vi "menu options.vi"(8 "error in":errorcluster, 9 "VI ref":refnum<vi>, 11 "menu ref in":refnum<k9>) -> (0 "error out":errorcluster, 3 "menu ref out":refnum<k9>)   [LabVIEW 2013, in "Standard Editor.lvlib"]
uses:
  Standard Editor.lvlib
  <vilib>/Utility/miscctls.llb/LVMenuShortCut.ctl
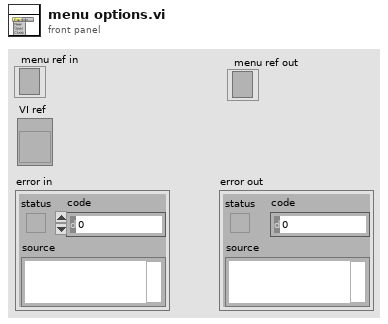
[diagram p1: front panel]
types:
  T1 = typedef "LVMenuShortCut.ctl" = cluster{"Include Shift Key?":bool, "Include Ctrl Key?":bool, "Shortcut Key":string}
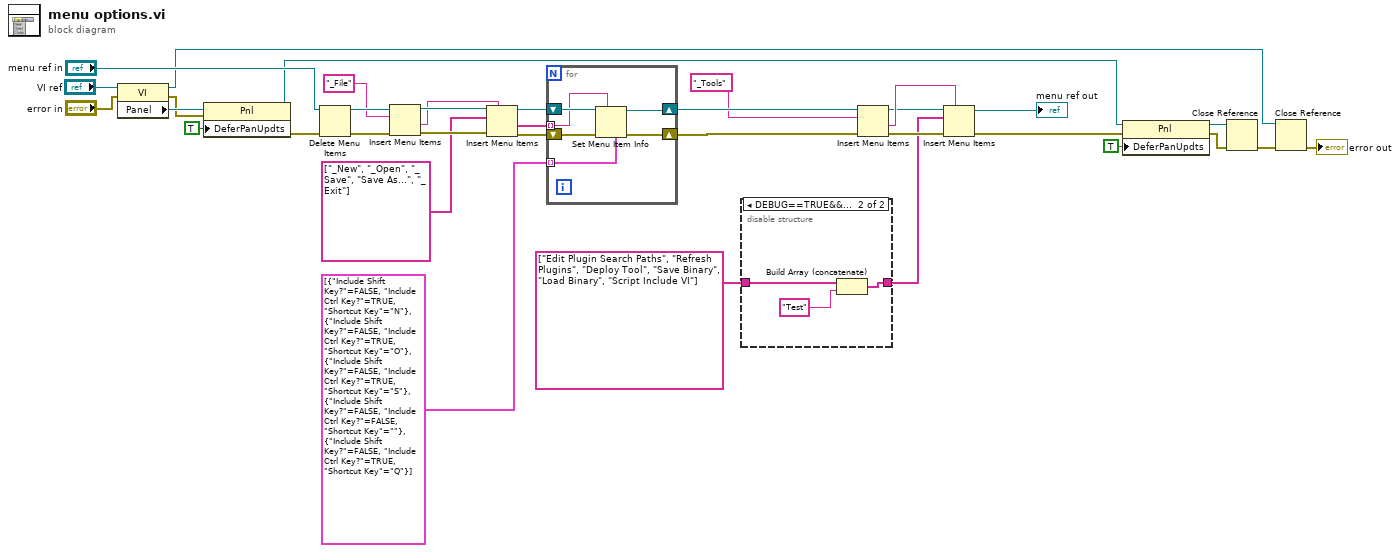
[diagram p0: block diagram]
diagram:
  n1 = property class="VI"(reference="VI ref", error in="error in") -> (reference out=w15:refnum<vi>, error out=w11:errorcluster, "Panel"=w14:refnum<vi>)
  n2 = property class="Pnl"(reference=w14, error in=w11, "DeferPanUpdts"=TRUE ("Defer Panel Updates")) -> (reference out=w7:refnum<vi>, error out=w10:errorcluster)
  n3 = Delete Menu Items(6:w10, 9:"menu ref in") -> (0:w30:errorcluster, 3:w34:refnum<k9>)  [unwired: 2 in]
  n4 = Insert Menu Items(6:w30, 8:"_File", 9:w34) -> (0:w29:errorcluster, 1:w31:string, 3:w32:refnum<k9>)  [unwired: 3 in]
  n5 = Insert Menu Items(5:w31, 6:w29, 8:string[] ["_New", "_Open", "_Save", "Save As...", "_Exit"] ("item names"), 9:w32) -> (0:w26:errorcluster, 1:w25:string[], 3:w27:refnum<k9>)  [unwired: 2 in]
  n6 = for {
    shift-right: [w39] -> w22
    shift-left: w27 -> [w41]
    tunnel: w25 -> [w38] mode=indexing
    tunnel: T1[] [{"Include Shift Key?"=FALSE, "Include Ctrl Key?"=TRUE, "Shortcut Key"="N"}, {"Include Shift Key?"=FALSE, "Include Ctrl Key?"=TRUE, "Shortcut Key"="O"}, {"Include Shift Key?"=FALSE, "Include Ctrl Key?"=TRUE, "Shortcut Key"="S"}, {"Include Shift Key?"=FALSE, "Include Ctrl Key?"=FALSE, "Shortcut Key"=""}, {"Include Shift Key?"=FALSE, "Include Ctrl Key?"=TRUE, "Shortcut Key"="Q"}] -> [w36] mode=indexing
    shift-right: [w37] -> w21
    shift-left: w26 -> [w40]
    n7 = Set Menu Item Info(4:w36, 7:w38, 8:w40, 11:w41) -> (0:w37:errorcluster, 3:w39:refnum<k9>)  [unwired: 3 in]
  }
  n8 = disable-structure shown="DEBUG==TRUE&&RUN_TIME_ENGINE==False" {
    disable-tunnel: [w42 w44] -> w2
    disable-tunnel: string[] ["Edit Plugin Search Paths", "Refresh Plugins", "Deploy Tool", "Save Binary", "Load Binary", "Script Include VI"] ("item names") -> [w42 w45]
    frame condition #0 {
    }
    frame condition #1 (active) {
      n9 = Build Array (concatenate)(w45, "Test") -> (w44:string[])
    }
  }
  n10 = Insert Menu Items(6:w21, 8:"_Tools", 9:w22) -> (0:w19:errorcluster, 1:w20:string, 3:w18:refnum<k9>)  [unwired: 3 in]
  n11 = Insert Menu Items(5:w20, 6:w19, 8:w2, 9:w18) -> (0:w8:errorcluster, 3:→"menu ref out":refnum<k9>)  [unwired: 2 in, 1 out]
  n12 = property class="Pnl"(reference=w7, error in=w8, "DeferPanUpdts"=TRUE ("Defer Panel Updates")) -> (reference out=w6:refnum<vi>, error out=w5:errorcluster)
  n13 = Close Reference(reference=w6, error in (no error)=w5) -> (error out=w4:errorcluster)
  n14 = Close Reference(reference=w15, error in (no error)=w4) -> (error out=→"error out":errorcluster)
